vi "Destroy.vi"(8 "error in (no error)":errorcluster, 10 "Shared Key":string, 11 "SMO":refnum<class "SMO.lvclass">) -> (0 "error out":errorcluster)   [LabVIEW 2013, in "SMO.lvclass"]
doc: "Destructor\n\nNote 01: This method is overridable by descendant\nNote 02: When overridden, Call Parent Method is required\n\n---------------------------------------------------------------\nJKI State Machine Objects™\nhttp://jki.net/state-machine-objects/\nCopyright (C) 2005-2015, JKI <info@jki.net>\nALL RIGHTS RESERVED"
uses:
  SMO.lvclass
  Registry/Registry-SMO.lvclass
panel:
  # "For instructions on how to use the JKI State Machine Objects, examples and video tutorials, visit:\nhttp://jki.net/state-machine-objects/\n\nJKI State Machine Objects™\nhttp://jki.net/state-machine-objects/\nCopyright (C) 2005-2015, JKI <info@jki.net>\nALL RIGHTS RESERVED"
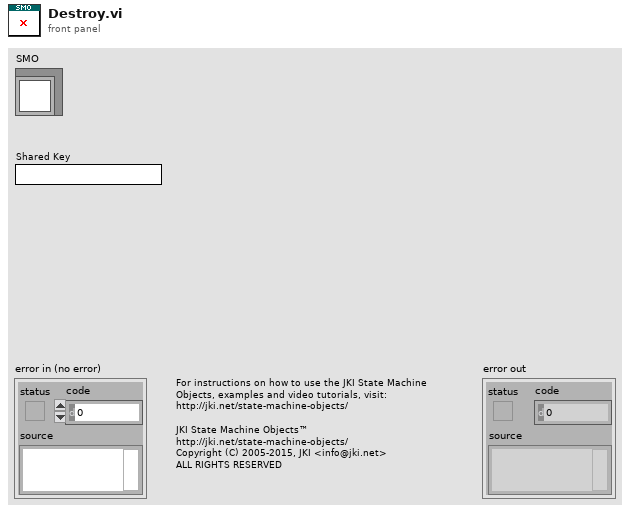
[diagram p1: front panel]
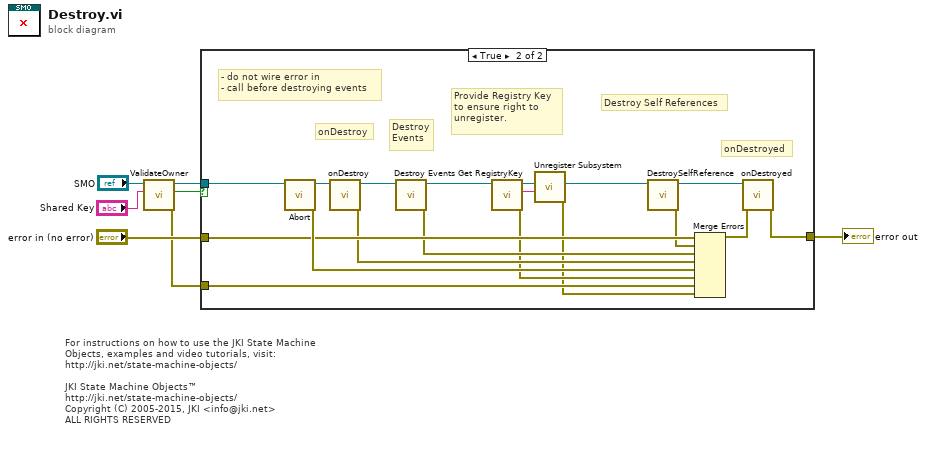
[diagram p0: block diagram]
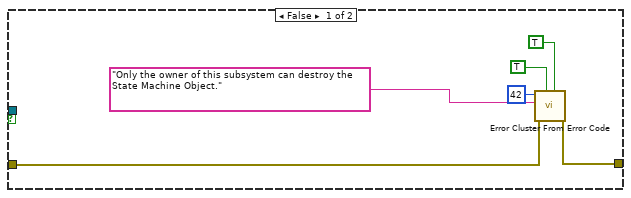
[diagram p2: hidden frame]
diagram:
  # "For instructions on how to use the JKI State Machine Objects, examples and video tutorials, visit:\nhttp://jki.net/state-machine-objects/\n\nJKI State Machine Objects™\nhttp://jki.net/state-machine-objects/\nCopyright (C) 2005-2015, JKI <info@jki.net>\nALL RIGHTS RESERVED"
  n1 = call "ValidateOwner.vi"("Shared Key"="Shared Key", "SMO in"="SMO") -> ("error out"=w2:errorcluster, "key matched"=w1:bool, "SMO out"=w4:refnum<class "SMO.lvclass">)  [unwired: 7 in]
  n2 = case shown="True" w1 {
    tunnel: "error in (no error)" -> [w10 w30]
    tunnel: [w9 w28] -> w6
    tunnel: w4 -> [_ w18]
    tunnel: w2 -> [_ w27]
    frame False {
      n3 = call <vilib>:"Error Cluster From Error Code.vi"("is warning? (False)"=TRUE, "show call chain? (False)"=TRUE, "error in (no error)"=w10, "error message (\"\")"="Only the owner of this subsystem can destroy the State Machine Object." ("error message (\"\")"), "error code (0)"=42) -> ("error out"=w9:errorcluster)  [unwired: 4 in]
    }
    frame True {
      # "Provide Registry Key\nto ensure right to \nunregister."
      # "Destroy\nEvents"
      # "Destroy Self References"
      # "onDestroy"
      # "onDestroyed"
      # "- do not wire error in\n- call before destroying events"
      n4 = call "Abort.vi"("SMO"=w18) -> ("error out"=w31:errorcluster, "SMO out"=w24:refnum<class "SMO.lvclass">)  [unwired: 9 in]
      n5 = call-dynamic "onDestroy.vi"("SMO"=w24) -> ("error out"=w22:errorcluster, "SMO out"=w23:refnum<class "SMO.lvclass">)  [unwired: 9 in]
      n6 = call "Destroy Events.vi"("SMO"=w23) -> ("error out"=w21:errorcluster, "SMO out"=w17:refnum<class "SMO.lvclass">)  [unwired: 9 in]
      n7 = call "Get RegistryKey.vi"("SMO"=w17) -> ("error out"=w16:errorcluster, "RegistryKey"=w19:string, "SMO out"=w20:refnum<class "SMO.lvclass">)  [unwired: 8 in]
      n8 = call "Unregister Subsystem.vi"("RegistryKey"=w19, "JKI SMO"=w20) -> ("error out"=w15:errorcluster, "JKI SMO out"=w14:refnum<class "SMO.lvclass">)  [unwired: 8 in]
      n9 = call-dynamic "DestroySelfReference.vi"("SMO"=w14) -> ("error out"=w25:errorcluster, "SMO out"=w26:refnum<class "SMO.lvclass">)  [unwired: 9 in]
      n10 = Merge Errors(w30, w25, w21, w22, w31, w16, w27, w15) -> (w29:errorcluster)
      n11 = call-dynamic "onDestroyed.vi"("error in (no error)"=w29, "SMO"=w26) -> ("error out"=w28:errorcluster)  [unwired: 9 in]
    }
  }
  "error out" <- w6
